vi "Conan Test.vi"   [LabVIEW 2018]
uses:
  Support/labview_conan_poc_liba.lvlibp
  Support/labview_conan_poc_libb.lvlibp
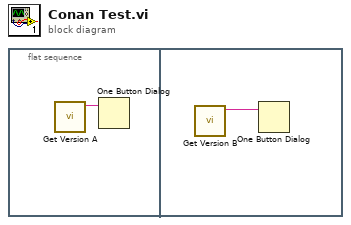
[diagram p0: block diagram]
diagram:
  n1 = flat-sequence {
    frame #0 {
      n2 = call "Get Version A.vi"() -> ("Version Out"=w1:string)  [unwired: 11 in]
      n3 = One Button Dialog(message=w1) -> ()  [unwired: 1 in, 1 out]
    }
    frame #1 {
      n4 = call "Get Version B.vi"() -> ("Version Out"=w2:string)  [unwired: 11 in]
      n5 = One Button Dialog(message=w2) -> ()  [unwired: 1 in, 1 out]
    }
  }
